vi "qWSL.vi"(0 "System no.":i32=1 min=1 max=4 step=1, 2 "Generator ID":i32[](array[numeric]) min=1 step=1, 3 "All generators?":bool, 5 "error in":errorcluster) -> (14 "WaveTable ID":i32[](array[numeric]), 19 "error out":errorcluster)   [LabVIEW 2026]
doc: "Returns current setting of wave table selection. If WaveTableID is zero no wave table is connected to the generator.\n\nC-413: Generator ID can be 1 to 2.\n\nC-886: Generator ID can be 1 to No. of connected axes.\n\nC-887: Generator ID can be 1 to No. of connected axes.\n\nC-891: Generator ID can be 1.\n\nE-709: Generator ID can be 1\n\nE-517: Generator ID can be 1 to 3. \n\nE-51: Generator ID can be 1 to 3. \n\nE-712: Generator ID can be 1 to No. of connected axes\n\nE-725, E-727: Generator ID can be 1 to No. of connected axes\n\nE-753: Generator ID can be 1\n\nE-754: Generator ID can be 1"
panel:
  # "Returns current setting of wave table selection."
  # "Query"
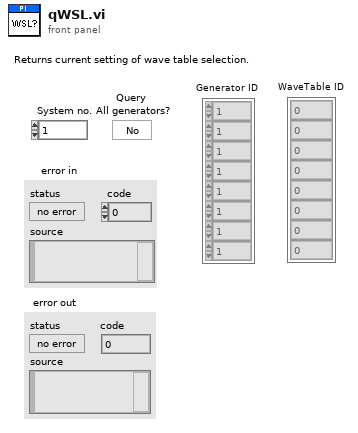
[diagram p1: front panel]
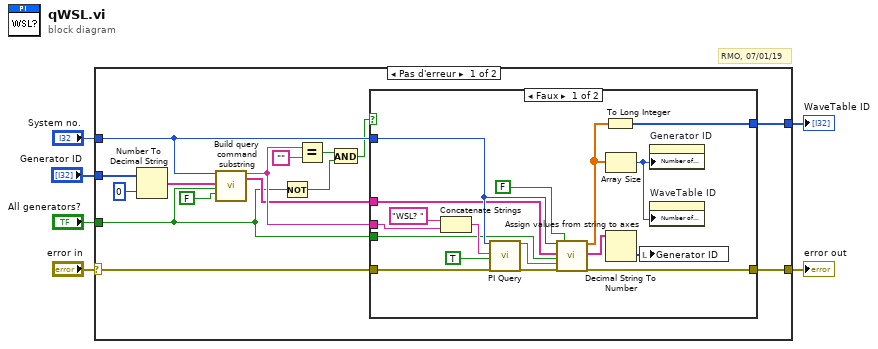
[diagram p0: block diagram]
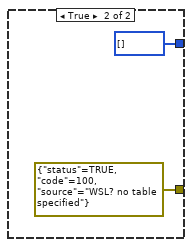
[diagram p2: hidden frame]
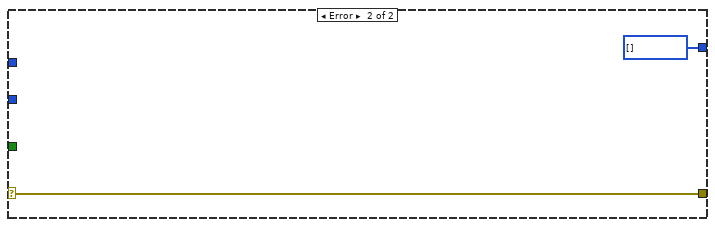
[diagram p3: hidden frame]
diagram:
  # "RMO, 07/01/19"
  n1 = case shown="Pas d'erreur" "error in" {
    selector: "error in" -> [w9 w41]
    tunnel: [w10 i32[] [] ("Values")] -> w6
    tunnel: "Generator ID" -> [w12 _]
    tunnel: [w8 w41] -> w4
    tunnel: "System no." -> [w19 _]
    tunnel: "All generators?" -> [w14 _]
    frame No Error {
      n2 = Number To Decimal String(number=w12, width (-)=i16 0) -> (decimal integer string=w11:string[])
      n3 = call "Build query command substring.vi"("System no."=w19, "Axes to query in"=w11, "Query\nAll axes?"=w14, "For all axes: use\nAxis identifier?"=FALSE ("For all axes: use\nAxis identifier?")) -> ("Command substring"=w20:string, "Axes to query out"=w18:string[])  [unwired: 2 in, 12 out]
      n4 = Not(x=w14) -> (.not. x?=w17:bool)
      n5 = Equal?(x=w20, y="" ("x")) -> (x = y?=w16:bool)
      n6 = And(x=w16, y=w17) -> (x .and. y?=w7:bool)
      n7 = case shown="Faux" w7 {
        tunnel: w20 -> [w35 _]
        tunnel: w19 -> [w34 _]
        tunnel: w18 -> [w33 _]
        tunnel: w14 -> [w30 _]
        tunnel: [w26 i32[] []] -> w10
        tunnel: w9 -> [w25 _]
        tunnel: [w24 errorcluster {"status"=TRUE, "code"=100, "source"="WSL? no table specified"} ("error out")] -> w8
        frame False {
          n8 = Concatenate Strings("WSL? ", w35) -> (w36:string)
          n9 = call "PI Query.vi"("System no."=w34, "String to send"=w36, "Attach termination char.?"=TRUE ("Attach Linefeed?"), "error in"=w25) -> ("String read"=w22:string, "error out"=w23:errorcluster)  [unwired: 3 in, 11 out]
          n10 = call "Assign values from string to axes.vi"("System no."=w34, "Queried axes"=w33, "All axes queried?"=w30, "Input String"=w22, "error in"=w23, "Axes related?"=FALSE) -> ("Values"=w32:dbl[], "Queried axes out"=w28:string[], "error out"=w24:errorcluster)  [unwired: 3 in, 8 out]
          n11 = To Long Integer(number=w32) -> (32bit integer=w26:i32[])
          n12 = Array Size(array=w32) -> (size(s)=w29:i32)
          n13 = Decimal String To Number(string=w28) -> (number=w27:i32[])  [unwired: 3 out]
          n14 = local write "Generator ID"(w27) -> ()
          n15 = property on="Generator ID" class="Tabl (strict)"("Number of Rows"=w29) -> ()  [unwired: 2 in, 2 out]
          n16 = property on="WaveTable ID" class="Tabl (strict)"("Number of Rows"=w29) -> ()  [unwired: 2 in, 2 out]
        }
        frame True {
        }
      }
    }
    frame Error {
    }
  }
  "error out" <- w4
  "WaveTable ID" <- w6
